vi "WebServiceLoop.vi"(8 "Error In":errorcluster, 11 "Message Queues":T1) -> (0 "Error Out":errorcluster)   [LabVIEW 2017, in "Server.lvlib" / "WebServiceCommunication.lvlib"]
doc: "This Loop sets, reads and calls the WebServiceFGV.vi which is responsible for communicating with the Webservice Methods.\nThis Loop has a timeout on the queue read function and will call the \"CheckClients\"-mode of the FGV frequently to validate which clients are still sending their heartbeat.\nIt is waiting for Messages in the WebServ-Queue and forwards messages (such as current clients connected to the MHL)."
uses:
  WebServiceCommunication.lvlib
  Message Queue/CommReferences.ctl
  Message Queue/MessageCluster.ctl
  WebServiceLoopData.ctl
  WebServiceFGVcommands.ctl
  TypeDefs/SR List.ctl
  TypeDefs/SR Data.ctl
  TypeDefs/ServerINI.ctl
  Oracle/OracleData.ctl
  <vilib>/Utility/error.llb/Error Cluster From Error Code.vi
  Message Queue/EnqueueMessage(Single).vi
  <vilib>/ErrorRing/Error Ring.xnode
  Message Queue/Message Queue.lvlib
  Server.lvlib
  ErrorLogger/ErrorLogger.lvlib
  Oracle/Oracle.lvlib
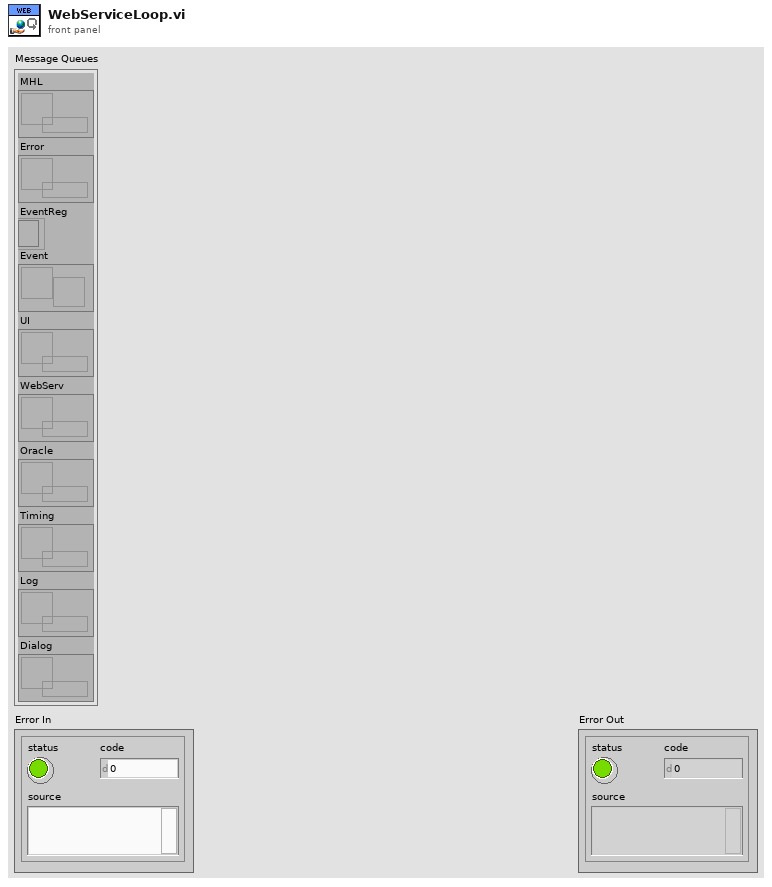
[diagram p1: front panel]
types:
  T1 = typedef "Server.lvlib/Message Queue.lvlib/CommReferences.ctl" = cluster{"MHL":refnum<queue>, "Error":refnum<queue>, "EventReg":refnum<event-registration>, "Event":refnum<user-event>, "UI":refnum<queue>, "WebServ":refnum<queue>, "Oracle":refnum<queue>, "Timing":refnum<queue>, "Log":refnum<queue>, "Dialog":refnum<queue>}
  T2 = typedef "Server.lvlib/WebServiceCommunication.lvlib/WebServiceLoopData.ctl" = cluster{"ClientTimeout":u32}
  T3 = typedef "Server.lvlib/ServerINI.ctl" = cluster{"ClientTimeout (s)":u32, "LogPath":path, "ErrorsToIgnore":i32[], "OracleData":T4}
  T4 = typedef "Server.lvlib/Oracle.lvlib/OracleData.ctl" = cluster{"DBname":string, "User":string, "Password":string}
  T5 = typedef "Server.lvlib/WebServiceCommunication.lvlib/WebServiceFGVcommands.ctl" = enum16{"Init", "Reset", "Heartbeat", "GetSRs", "SetSRs", "CheckClients", "GetClients"}
  T6 = typedef "Server.lvlib/SR List.ctl" = T7[]
  T7 = typedef "Server.lvlib/SR Data.ctl" = cluster{"SR#":dbl, "Group":string, "Owner":string, "Problem Summary":string, "Last Updated":timestamp, "Customer First Name":string, "Customer Last Name":string, "Company":string, "Created On":timestamp, "SR Type":string, "Status":string, "Service Level":string, "Channel":string, "Days Open":dbl}
  T8 = typedef "Server.lvlib/ClientList.ctl" = T9[]
  T9 = typedef "Server.lvlib/ClientData.ctl" = cluster{"ClientID":string, "LastHeartbeat":timestamp}
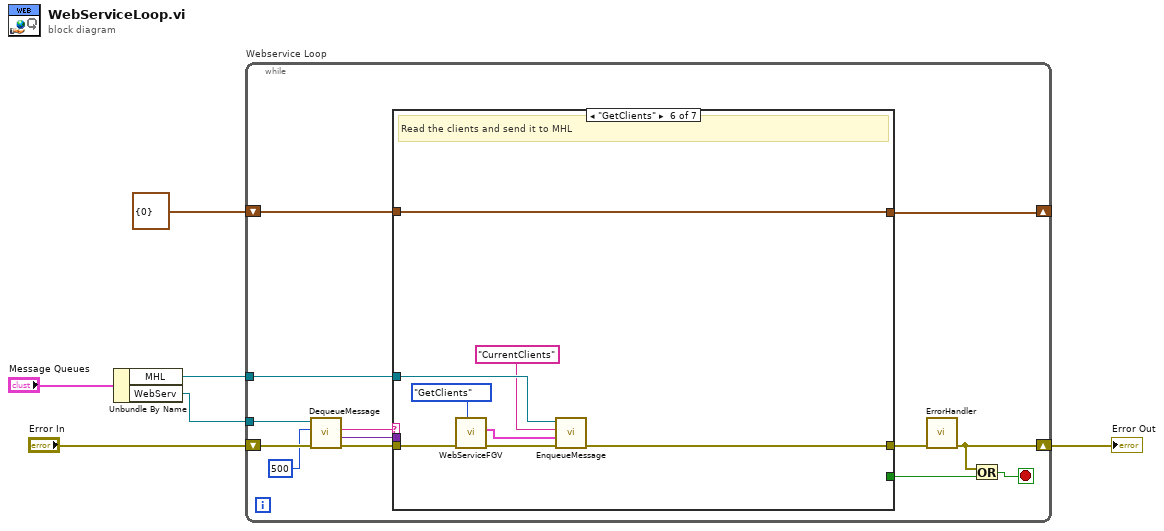
[diagram p0: block diagram]
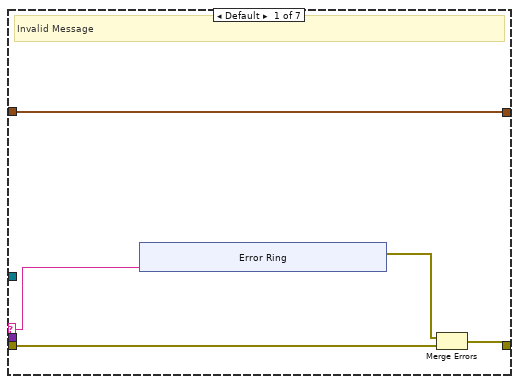
[diagram p2: hidden frame]
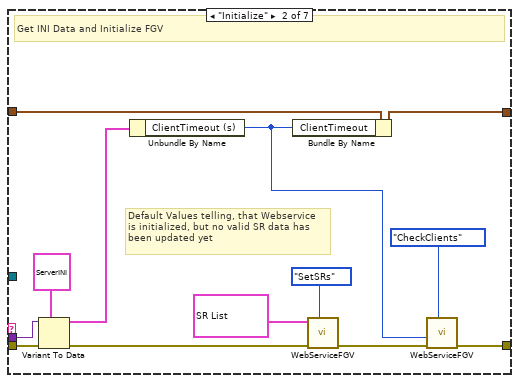
[diagram p3: hidden frame]
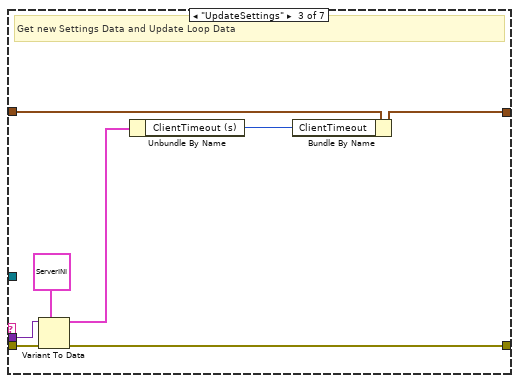
[diagram p4: hidden frame]
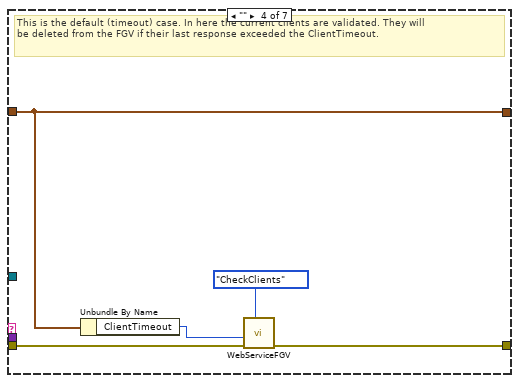
[diagram p5: hidden frame]
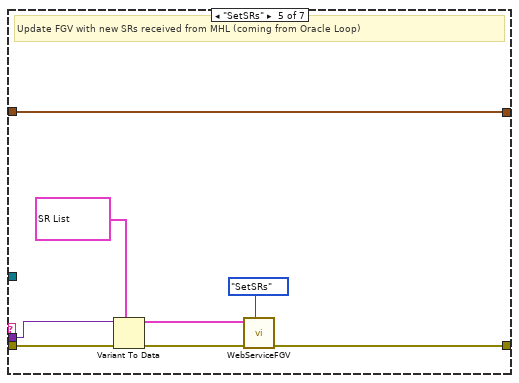
[diagram p6: hidden frame]
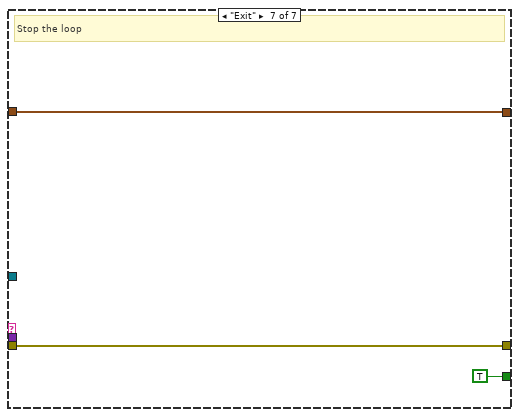
[diagram p7: hidden frame]
diagram:
  n1 = Unbundle By Name("Message Queues") -> ("MHL"=w2:refnum<queue>, "WebServ"=w3:refnum<queue>)
  n2 = while "Webservice Loop" {
    shift-right: [w7] -> w5
    shift-left: "Error In" -> [w19]
    tunnel: w3 -> [w16]
    tunnel: w2 -> [w11]
    shift-right: [w9] -> _
    shift-left: T2 {"ClientTimeout"=0} ("WebServiceLoopData") -> [w10]
    stop <- w8 stop-if-true
    n3 = call "DequeueMessage.vi"("error in (no error)"=w19, "timeout ms (-1)"=500, "Message Queue"=w16) -> ("error out"=w17:errorcluster, "Message Data"=w14:variant, "Message"=w15:string)  [unwired: 4 in, 2 out]
    n4 = case shown="\"GetClients\"" w15 {
      selector: w15 -> [w21 _ _ _ _ _ _]
      tunnel: [w23 w40 w50 w56 w64 w70 w76] -> w18
      tunnel: w17 -> [w24 w44 w52 w57 w65 w73 w76]
      tunnel: w14 -> [_ w35 w48 _ w62 _ _]
      tunnel: [_ _ _ _ _ _ TRUE] -> w13
      tunnel: w11 -> [_ _ _ _ _ w69 _]
      tunnel: [w20 w34 w47 w54 w58 w66 w74] -> w9
      tunnel: w10 -> [w20 w38 w51 w54 w58 w66 w74]
      frame Default {
        # "Invalid Message"
        n5 = xnode "Error Ring"("parameter 0"=w21) -> ("error out"=w22:errorcluster)
        n6 = Merge Errors(w22, w24) -> (w23:errorcluster)
      }
      frame "Initialize" {
        # "Default Values telling, that Webservice\nis initialized, but no valid SR data has\nbeen updated yet"
        # "Get INI Data and Initialize FGV"
        n7 = Variant To Data(error in=w44, type=T3 {"ClientTimeout (s)"=30, "LogPath"=path "C:/Users/jgoebel/Documents/GitHub/AEDashboard/ServerLib/Data/ServerLog.tdms", "ErrorsToIgnore"=[], "OracleData"={"DBname"="", "User"="", "Password"=""}} ("ServerINI"), Variant=w35) -> (data=w33:T3, error out=w37:errorcluster)
        n8 = Unbundle By Name(w33) -> ("ClientTimeout (s)"=w32:u32)
        n9 = Bundle By Name(cluster=w38, "ClientTimeout"=w32) -> (w34:T2)
        n10 = call "WebServiceFGV.vi"("CMD"=WebServiceFGVcommands."SetSRs", "error in (no error)"=w37, "SRListIn"=T6 [{"SR#"=1234.0, "Group"="THIS IS A DUMMY SR!", "Owner"="WEBSERVER IS INITIALIZED!", "Problem Summary"="BUT NO VALID SR DATA IS SET YET!", "Last Updated"=timestamp(0 s since 1904-01-01), "Customer First Name"="", "Customer Last Name"="", "Company"="", "Created On"=timestamp(0 s since 1904-01-01), "SR Type"="", "Status"="", "Service Level"="", "Channel"="", "Days Open"=0.0}]) -> ("error out"=w41:errorcluster)  [unwired: 6 in, 2 out]
        n11 = call "WebServiceFGV.vi"("CMD"=WebServiceFGVcommands."CheckClients", "error in (no error)"=w41, "ClientTimeout(s)(30)"=w32) -> ("error out"=w40:errorcluster)  [unwired: 6 in, 2 out]
      }
      frame "UpdateSettings" {
        # "Get new Settings Data and Update Loop Data"
        n12 = Variant To Data(error in=w52, type=T3 {"ClientTimeout (s)"=30, "LogPath"=path "C:/Users/jgoebel/Documents/GitHub/AEDashboard/ServerLib/Data/ServerLog.tdms", "ErrorsToIgnore"=[], "OracleData"={"DBname"="", "User"="", "Password"=""}} ("ServerINI"), Variant=w48) -> (data=w46:T3, error out=w50:errorcluster)
        n13 = Unbundle By Name(w46) -> ("ClientTimeout (s)"=w45:u32)
        n14 = Bundle By Name(cluster=w51, "ClientTimeout"=w45) -> (w47:T2)
      }
      frame "" {
        # "This is the default (timeout) case. In here the current clients are validated. They will\nbe deleted from the FGV if their last response exceeded the ClientTimeout."
        n15 = Unbundle By Name(w54) -> ("ClientTimeout"=w53:u32)
        n16 = call "WebServiceFGV.vi"("CMD"=WebServiceFGVcommands."CheckClients", "error in (no error)"=w57, "ClientTimeout(s)(30)"=w53) -> ("error out"=w56:errorcluster)  [unwired: 6 in, 2 out]
      }
      frame "SetSRs" {
        # "Update FGV with new SRs received from MHL (coming from Oracle Loop)"
        n17 = Variant To Data(error in=w65, type=T6 [{"SR#"=0.0, "Group"="", "Owner"="", "Problem Summary"="", "Last Updated"=timestamp(0 s since 1904-01-01), "Customer First Name"="", "Customer Last Name"="", "Company"="", "Created On"=timestamp(0 s since 1904-01-01), "SR Type"="", "Status"="", "Service Level"="", "Channel"="", "Days Open"=0.0}] ("SRListIn"), Variant=w62) -> (data=w60:T6, error out=w63:errorcluster)
        n18 = call "WebServiceFGV.vi"("CMD"=WebServiceFGVcommands."SetSRs", "error in (no error)"=w63, "SRListIn"=w60) -> ("error out"=w64:errorcluster)  [unwired: 6 in, 2 out]
      }
      frame "GetClients" {
        # "Read the clients and send it to MHL"
        n19 = call "WebServiceFGV.vi"("CMD"=WebServiceFGVcommands."GetClients", "error in (no error)"=w73) -> ("error out"=w72:errorcluster, "ClientList"=w67:T8)  [unwired: 7 in, 1 out]
        n20 = call-poly "EnqueueMessage.vi"("error in (no error)"=w72, "Message Data"=w67, "Message"="CurrentClients", "Message Queue"=w69) -> ("error out"=w70:errorcluster)  [unwired: 6 in, 1 out]
      }
      frame "Exit" {
        # "Stop the loop"
      }
    }
    n21 = call "ErrorHandler.vi"("error in (no error)"=w18) -> ("error out"=w7:errorcluster)  [unwired: 10 in]
    n22 = Or(x=w7, y=w13) -> (x .or. y?=w8:bool)
  }
  "Error Out" <- w5
